vi "Get Class Hierarchy.vi"(8 "error in (no error)":errorcluster, 11 "Base Class Name":string) -> (0 "error out":errorcluster, 1 "Success?":bool, 3 "Class Hierarchy":string[](array[string]))   [LabVIEW 2019, in "ClassLoader.lvlib"]
doc: "Return a map containing all the members for the given class.\n\nThis VI does not automatically load data. Front-load before calling this VI!"
uses:
  ClassLoader.lvlib
  <vilib>/Utility/config.llb/NI_LVConfig.lvlib
  Sub/Cache/Cache_Hierarchy Global.vi
  Sub/Ctl/Ctl_Hierarchy Cluster.ctl
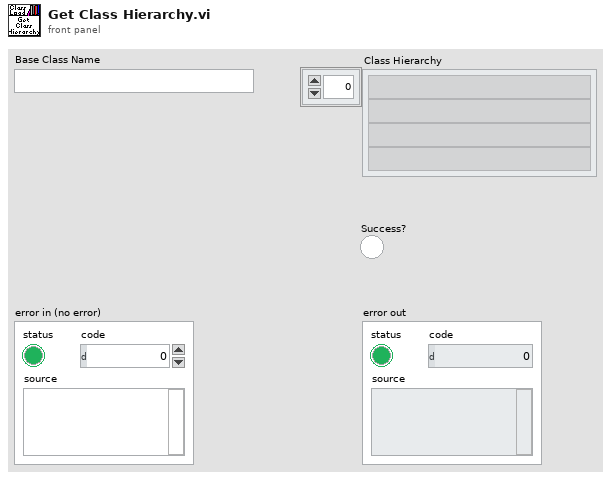
[diagram p1: front panel]
types:
  T1 = typedef "ClassLoader.lvlib/Ctl_Hierarchy Cluster.ctl" = cluster{"Hierarchy":string[]}
  T2 = typedef "NI_LVConfig.lvlib/Config Data RefNum.ctl" = refnum<k1>
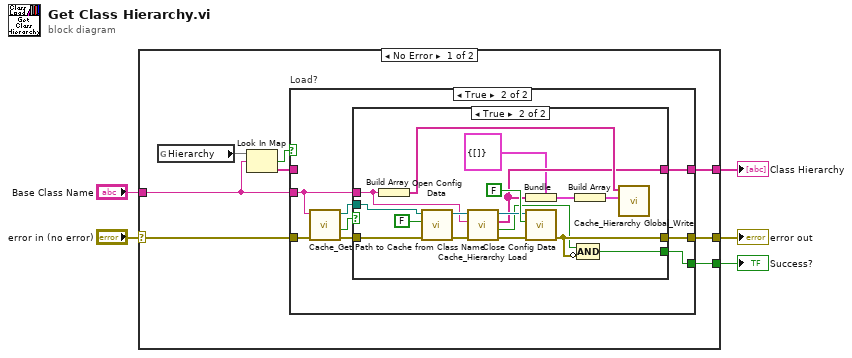
[diagram p0: block diagram]
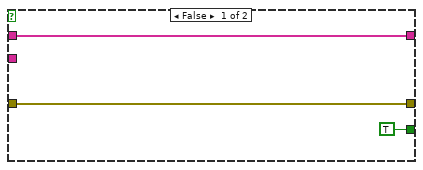
[diagram p2: hidden frame]
diagram:
  n1 = case shown="No Error" "error in (no error)" {
    selector: "error in (no error)" -> [w13 w43]
    tunnel: "Base Class Name" -> [w9 _]
    tunnel: [w12 w43] -> w3
    tunnel: [w11 _] -> w2
    tunnel: [w10 _] -> w1
    frame No Error {
      n2 = global read "Cache_Hierarchy Global.vi" "Hierarchy"() -> (w6:map{string, string[]})
      n3 = Look In Map(map=w6, key=w9) -> (key not found?=w8:bool, value=w7:string[])  [unwired: 1 in]
      n4 = case "Load?" shown="True" w8 {
        tunnel: w13 -> [w15 w24]
        tunnel: [w15 w20] -> w12
        tunnel: [TRUE w19] -> w11
        tunnel: [w16 w18] -> w10
        tunnel: w9 -> [_ w17]
        tunnel: w7 -> [w16 _]
        frame False {
        }
        frame True {
          n5 = call "Cache_Get Path to Cache from Class Name.vi"("error in (no error)"=w24, "Class Name"=w17) -> ("error out"=w21:errorcluster, "Success?"=w22:bool, "Cache Path"=w23:path)  [unwired: 7 in]
          n6 = case shown="True" w22 {
            tunnel: w23 -> [_ w40]
            tunnel: w17 -> [_ w31]
            tunnel: w21 -> [w25 w39]
            tunnel: [w25 w38] -> w20
            tunnel: [_ w37] -> w19
            tunnel: [_ w29] -> w18
            frame False {
            }
            frame True {
              n7 = Build Array(w31) -> (w30:string[])
              n8 = call <vilib>:"Open Config Data.vi"("error in (no error)"=w39, "create file if necessary (T)"=FALSE, "configuration file path"=w40) -> ("error out"=w33:errorcluster, "refnum"=w36:T2)  [unwired: 6 in, 1 out]
              n9 = call "Cache_Hierarchy Load.vi"("error in (no error)"=w33, "Class Name"=w31, "Refnum in"=w36) -> ("error out"=w32:errorcluster, "Success?"=w34:bool, "Hierarchy"=w29:string[], "Refnum out"=w35:T2)  [unwired: 5 in]
              n10 = Bundle(cluster=T1 {"Hierarchy"=[]} ("Hierarchy Cluster"), "Hierarchy"=w29) -> (w28:T1)
              n11 = call <vilib>:"Close Config Data.vi"("error in (no error)"=w32, "write file if changed (T)"=FALSE, "refnum"=w35) -> ("error out"=w38:errorcluster)  [unwired: 7 in, 1 out]
              n12 = Build Array(w28) -> (w26:T1[])
              n13 = Compound Arithmetic op=AND(w34, invert w38) -> (w37:bool)
              n14 = call "Cache_Hierarchy Global_Write.vi"("Class Hierarchies"=w26, "Class Names"=w30) -> ()  [unwired: 9 in, 1 out]
            }
          }
        }
      }
    }
    frame Error {
    }
  }
  "error out" <- w3
  "Success?" <- w2
  "Class Hierarchy" <- w1
